vi "FRANCELINO_VI02.vi"() -> ()   [LabVIEW 2018]
panel:
  out "Boolean 4":bool
  out "Boolean 3":bool
  out "Boolean 2":bool
  out "Boolean":bool
  in  "Z":dbl(slide) scale=-2.0..2.0
  in  "Y":dbl(slide) scale=-2.0..2.0
  in  "X":dbl(slide) scale=-2.0..2.0
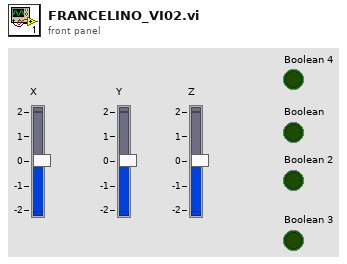
[diagram p1: front panel]
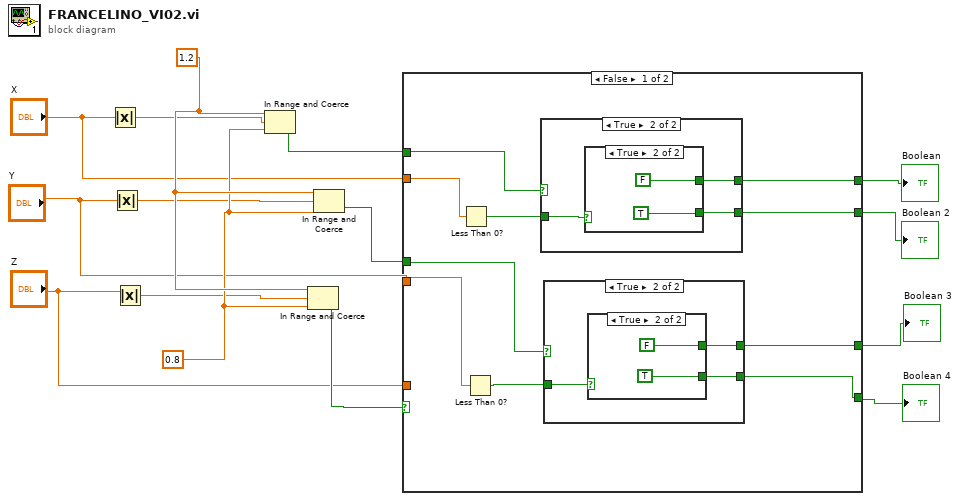
[diagram p0: block diagram]
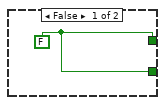
[diagram p2: hidden frame]
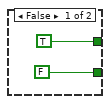
[diagram p3: hidden frame]
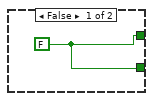
[diagram p4: hidden frame]
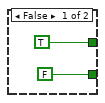
[diagram p5: hidden frame]
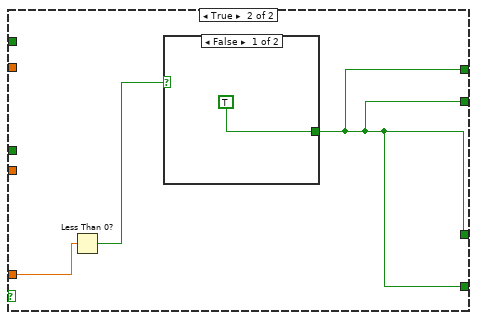
[diagram p6: hidden frame]
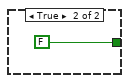
[diagram p7: hidden frame]
diagram:
  w14 = 0.8
  w15 = 1.2
  n1 = Absolute Value(x="X") -> (abs(x)=w13:dbl)
  n2 = Absolute Value(x="Y") -> (abs(x)=w12:dbl)
  n3 = Absolute Value(x="Z") -> (abs(x)=w11:dbl)
  n4 = In Range and Coerce(upper limit=w15, x=w13, lower limit=w14) -> (In Range?=w8:bool)  [unwired: 1 out]
  n5 = In Range and Coerce(upper limit=w15, x=w11, lower limit=w14) -> (In Range?=w10:bool)  [unwired: 1 out]
  n6 = In Range and Coerce(upper limit=w15, x=w12, lower limit=w14) -> (In Range?=w9:bool)  [unwired: 1 out]
  n7 = case shown="False" w10 {
    tunnel: "Y" -> [w25 _]
    tunnel: w9 -> [w24 _]
    tunnel: w8 -> [w23 _]
    tunnel: "X" -> [w22 _]
    tunnel: [w19 w42] -> w6
    tunnel: [w18 w42] -> w5
    tunnel: [w16 w42] -> w4
    tunnel: [w17 w42] -> w3
    tunnel: "Z" -> [_ w44]
    frame False {
      n8 = Less Than 0?(x=w22) -> (x < 0?=w20:bool)
      n9 = Less Than 0?(x=w25) -> (x < 0?=w21:bool)
      n10 = case shown="True" w23 {
        tunnel: w20 -> [_ w37]
        tunnel: [w34 w36] -> w19
        tunnel: [w34 w35] -> w18
        frame False {
          w34 = FALSE
        }
        frame True {
          n11 = case shown="True" w37 {
            tunnel: [TRUE FALSE] -> w36
            tunnel: [FALSE TRUE] -> w35
            frame False {
            }
            frame True {
            }
          }
        }
      }
      n12 = case shown="True" w24 {
        tunnel: w21 -> [_ w29]
        tunnel: [w26 w28] -> w17
        tunnel: [w26 w27] -> w16
        frame False {
          w26 = FALSE
        }
        frame True {
          n13 = case shown="True" w29 {
            tunnel: [FALSE TRUE] -> w27
            tunnel: [TRUE FALSE] -> w28
            frame False {
            }
            frame True {
            }
          }
        }
      }
    }
    frame True {
      n14 = Less Than 0?(x=w44) -> (x < 0?=w43:bool)
      n15 = case shown="False" w43 {
        tunnel: [TRUE FALSE] -> w42
        frame False {
        }
        frame True {
        }
      }
    }
  }
  "Boolean" <- w6
  "Boolean 2" <- w5
  "Boolean 3" <- w3
  "Boolean 4" <- w4
